vi "Correction Short Status Query.vi"(8 "error in (no error)":errorcluster, 11 "VISA resource name":refnum<visa-resource-name>) -> (0 "error out":errorcluster, 2 "Short Status":string, 3 "VISA resource name out":refnum<visa-resource-name>)   [LabVIEW 2014, in "LCR Meter.lvlib"]
doc: "Returns the SHORT correction function."
uses:
  <instrlib>/LCR Meter/Examples/LCR Meter Acquire Single_1 Folder/LCR Meter.lvlib
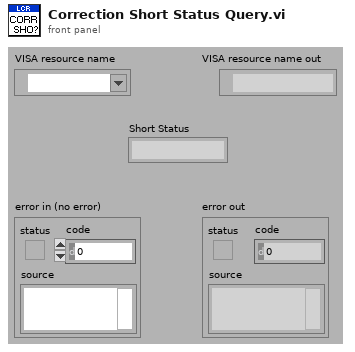
[diagram p1: front panel]
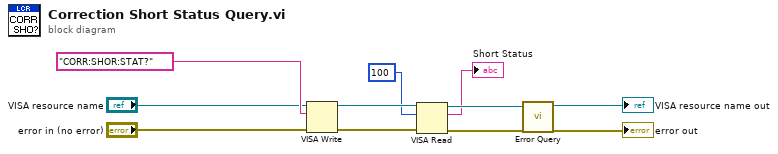
[diagram p0: block diagram]
diagram:
  n1 = VISA Write(VISA resource name="VISA resource name", write buffer="CORR:SHOR:STAT?", error in (no error)="error in (no error)") -> (VISA resource name out=w6:refnum<visa-resource-name>, error out=w4:errorcluster)  [unwired: 1 out]
  n2 = VISA Read(VISA resource name=w6, byte count=u32 100, error in (no error)=w4) -> (VISA resource name out=w5:refnum<visa-resource-name>, read buffer=→"Short Status":string, error out=w3:errorcluster)  [unwired: 1 out]
  n3 = call <instrlib>:"Error Query.vi"("error in (no error)"=w3, "VISA resource name"=w5) -> ("error out"=→"error out":errorcluster, "VISA resource name out"=→"VISA resource name out":refnum<visa-resource-name>)  [unwired: 6 in, 2 out]
